vi "DIO 입출력 설정관리.vi"() -> ()   [LabVIEW 2019]
panel:
  out "클러스터":cluster{"line grouping":i32, "lines":tag}={"line grouping"=1, "lines"=""} {"line grouping" items=["각 라인에 하나의 채널", "모든 라인에 하나의 채널"]}
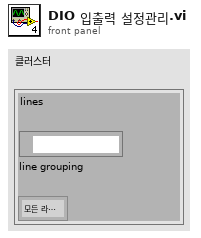
[diagram p1: front panel]
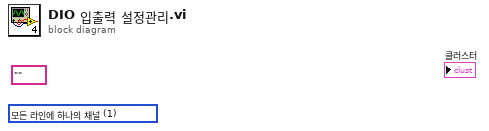
[diagram p0: block diagram]
diagram:
  w1 = 1 items=["각 라인에 하나의 채널", "모든 라인에 하나의 채널"] ("line grouping")
  w2 = tag "" ("lines")
